vi "Dynamic Scrollbars - Resize Front Panel.vi"(8 "error in":errorcluster, 9 "OrgBnds":T1, 10 "NewBnds":T1, 11 "VI Ref":refnum<vi>) -> (0 "error out":errorcluster, 3 "VI Ref":refnum<vi>)   [LabVIEW 2014]
doc: "<B>Copyright</B>: (c) 2015 MHWirth. All rights reserved.\n\nThis subVI dynamically enables/disables scrollbars when front panel size becomes smaller than the fixed front panel size. \n\nIt can be called in \"Panel Resize\" event VI when action is \"Resized\"."
uses:
  <vilib>/Utility/miscctls.llb/LVRectTypeDef.ctl
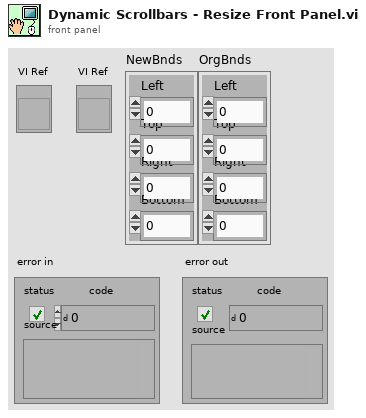
[diagram p1: front panel]
types:
  T1 = typedef "LVRectTypeDef.ctl" = cluster{"Left":i16, "Top":i16, "Right":i16, "Bottom":i16}
  T2 = enum16{"Always On", "Always Off", "Off While Running"}
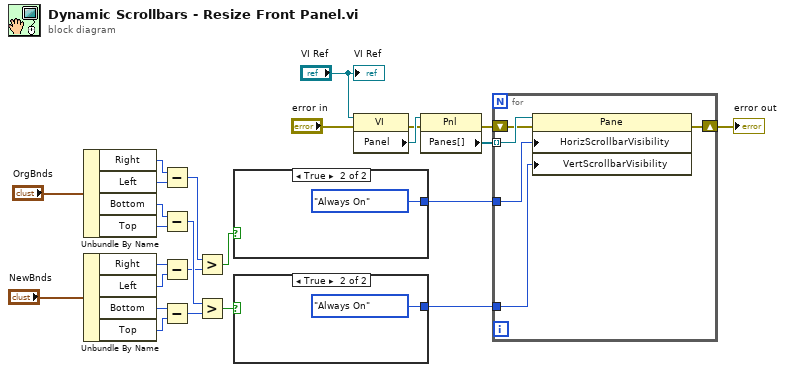
[diagram p0: block diagram]
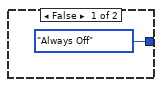
[diagram p2: hidden frame]
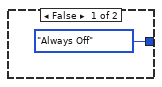
[diagram p3: hidden frame]
diagram:
  n1 = Unbundle By Name("OrgBnds") -> ("Right"=w13:i16, "Left"=w14:i16, "Bottom"=w15:i16, "Top"=w16:i16)
  n2 = Unbundle By Name("NewBnds") -> ("Right"=w12:i16, "Left"=w11:i16, "Bottom"=w10:i16, "Top"=w9:i16)
  n3 = Subtract(x=w13, y=w14) -> (x-y=w8:i16)
  n4 = Subtract(x=w15, y=w16) -> (x-y=w7:i16)
  n5 = Subtract(x=w12, y=w11) -> (x-y=w6:i16)
  n6 = Subtract(x=w10, y=w9) -> (x-y=w5:i16)
  n7 = Greater?(x=w8, y=w6) -> (0:w18:bool)
  n8 = Greater?(x=w7, y=w5) -> (0:w17:bool)
  n9 = case shown="True" w18 {
    tunnel: [T2."Always Off" ("Horizontal Scrollbar Visibility") T2."Always On" ("Horizontal Scrollbar Visibility")] -> w21
    frame False {
    }
    frame True {
    }
  }
  n10 = case shown="True" w17 {
    tunnel: [T2."Always Off" ("Horizontal Scrollbar Visibility") T2."Always On" ("Horizontal Scrollbar Visibility")] -> w20
    frame False {
    }
    frame True {
    }
  }
  n11 = property class="VI"(reference="VI Ref", error in="error in") -> (error out=w24:errorcluster, "Panel"=w25:refnum<vi>)  [unwired: 1 out]
  n12 = property class="Pnl"(reference=w25, error in=w24) -> (error out=w23:errorcluster, "Panes[]"=w22:refnum<vi>[])  [unwired: 1 out]
  n13 = for {
    shift-right: [w32] -> w3
    shift-left: w23 -> [w33]
    tunnel: w22 -> [w34] mode=indexing
    tunnel: w21 -> [w31]
    tunnel: w20 -> [w30]
    n14 = property class="Pane"(reference=w34, error in=w33, "HorizScrollbarVisibility"=w31, "VertScrollbarVisibility"=w30) -> (error out=w32:errorcluster)  [unwired: 1 out]
  }
  "error out" <- w3
  "VI Ref" <- "VI Ref"
